vi "scanDataView.vi"(10 "UserEvents in":refnum<class "UserEvents.lvclass">) -> ()   [LabVIEW 2015, in "FAMTViews.lvlib"]
uses:
  FAMTViews.lvlib
  UserEvents/UserEvents.lvclass
  UserEvents/UserEvents.lvclass/UserEvents.ctl
  Typedefs/StateSelector.ctl
  Typedefs/FAMTTypedefs.lvlib
panel:
  out "Pressure":dbl[unit] format="%.3f"
  out "Error":dbl format="%.3f"
  out "Actual Force":dbl[unit] format="%.3f"
  out "Current Demand":dbl format="%.3f"
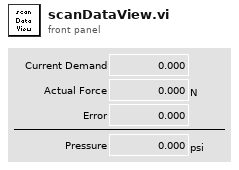
[diagram p1: front panel]
types:
  T1 = typedef "FAMTTypedefs.lvlib/PubDataEvents.ctl" = cluster{"State":refnum<user-event>, "ErrorCode":refnum<user-event>, "ADC Outputs":refnum<user-event>, "InputData":refnum<user-event>, "ControllerData":refnum<user-event>, "TestStatus":refnum<user-event>, "LogPath":refnum<user-event>, "ILC Outputs":refnum<user-event>, "Scan Progress":refnum<user-event>}
  T2 = cluster{"Event Registration Refnum":refnum<event-registration>, "Event Registration Refnum":refnum<event-registration>}
  T3 = typedef "FAMTTypedefs.lvlib/StateSelector.ctl" = enum16{"OfflineState", "FaultState", "StandbyState", "DisabledState", "EnabledState", "WaitForUserInputState", "PerformOpenLoopScanState", "PerformPreScanHoldState", "PerformPostScanHoldState", "PerformScanState"}
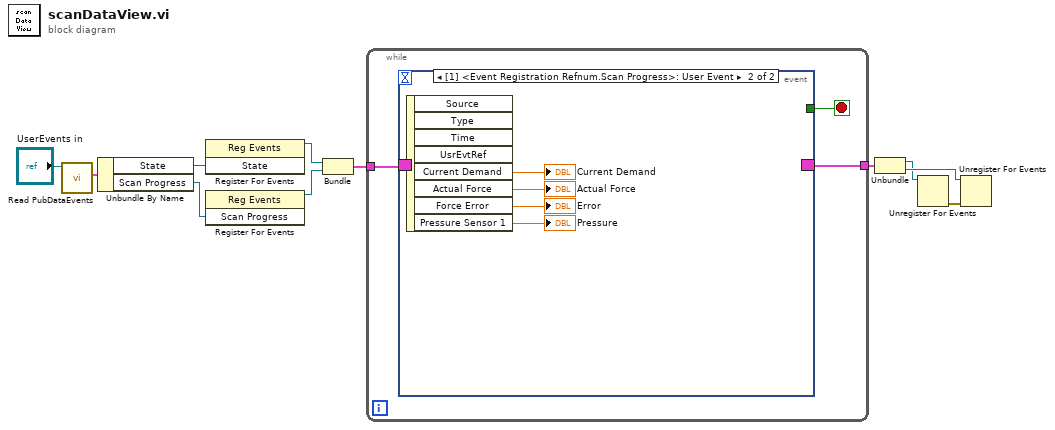
[diagram p0: block diagram]
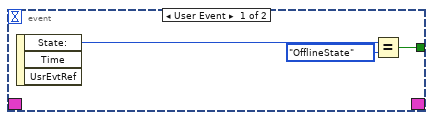
[diagram p2: hidden frame]
diagram:
  n1 = call "Read PubDataEvents.vi"("UserEvents in"="UserEvents in") -> ("PubDataEvents"=w10:T1)  [unwired: 9 in, 1 out]
  n2 = Unbundle By Name(w10) -> ("State"=w9:refnum<user-event>, "Scan Progress"=w11:refnum<user-event>)
  n3 = register-events(w9) -> (reference out=w7:refnum<event-registration>)  [unwired: 2 in, 1 out]
  n4 = register-events(w11) -> (reference out=w8:refnum<event-registration>)  [unwired: 2 in, 1 out]
  n5 = Bundle("Event Registration Refnum"=w7, "Event Registration Refnum"=w8) -> (w1:T2)  [unwired: 1 in]
  n6 = while {
    tunnel: [w14] -> w3
    tunnel: w1 -> [w12]
    stop <- w13 stop-if-true
    n7 = event shown="[1] <Event Registration Refnum.Scan Progress>: User Event" {
      selector: w12 -> [_ _]
      dyn-events: [_ _] -> w14
      timeout: _ -> [_ _]
      tunnel: [w16 _] -> w13
      event User Event {
        n8 = event-data() -> ("State:"=w15:T3)  [unwired: 1 in, 2 out]
        n9 = Equal?(x=w15, y=StateSelector."OfflineState") -> (x = y?=w16:bool)
      }
      event User Event {
        n10 = event-data() -> ("Current Demand"=→"Current Demand":dbl, "Actual Force"=→"Actual Force":dbl[unit], "Force Error"=→"Error":dbl, "Pressure Sensor 1"=→"Pressure":dbl[unit])  [unwired: 1 in, 4 out]
      }
    }
  }
  n11 = Unbundle(w3) -> ("Event Registration Refnum"=w2:refnum<event-registration>, "Event Registration Refnum"=w4:refnum<event-registration>)
  n12 = Unregister For Events(event registration refnum=w2) -> (error out=w5:errorcluster)  [unwired: 1 in]
  n13 = Unregister For Events(event registration refnum=w4, error in=w5) -> ()  [unwired: 1 out]
